vi "Unwrap Phase PtByPt.vi"(7 "initialize":bool, 10 "wrap base":dbl=6.283185307179586, 11 "phase":dbl format="%0.2f") -> (3 "unwrapped phase":dbl format="%0.2f")   [LabVIEW 2020, in "NI_PtbyPt.lvlib"]
doc: "Unwraps <B>phase</B> by eliminating discontinuities whose absolute values exceed half of <B>wrap base</B>."
uses:
  NI_PtbyPt.lvlib
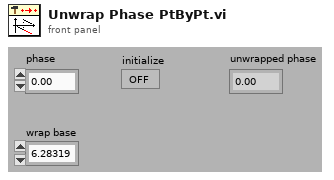
[diagram p1: front panel]
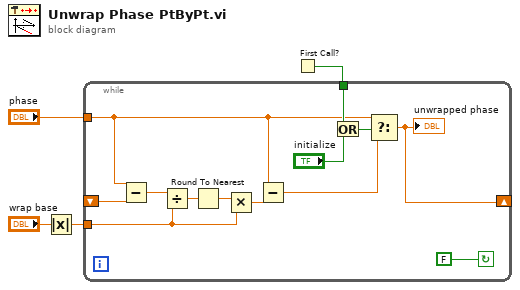
[diagram p0: block diagram]
diagram:
  n1 = Absolute Value(x="wrap base") -> (abs(x)=w1:dbl)
  n2 = First Call?() -> (First Call?: T/F=w4:bool)
  n3 = while {
    tunnel: w4 -> [w14]
    shift-left: _ -> [w17]
    shift-right: [w5] -> _
    tunnel: w1 -> [w7]
    tunnel: "phase" -> [w6]
    stop <- FALSE continue-if-true
    n4 = Subtract(x=w6, y=w17) -> (x-y=w12:dbl)
    n5 = Divide(x=w12, y=w7) -> (x/y=w11:dbl)
    n6 = Round To Nearest(number=w11) -> (nearest integer value=w10:dbl)
    n7 = Multiply(x=w10, y=w7) -> (x*y=w9:dbl)
    n8 = Subtract(x=w6, y=w9) -> (x-y=w8:dbl)
    n9 = Or(x=w14, y="initialize") -> (x .or. y?=w13:bool)
    n10 = Select(t=w6, s=w13, f=w8) -> (s? t:f=w5:dbl)
    "unwrapped phase" <- w5
  }
